vi "fgv_Acq Exited.vi"(8 "error in (no error)":errorcluster, 9 "Function":T1, 11 "Acquisition completed":bool) -> (0 "error out":errorcluster, 3 "Acquisition completed":bool)   [LabVIEW 2020]
uses:
  Typedefs/Read Write Enum.ctl
panel:
  # "SUBROUTINE"
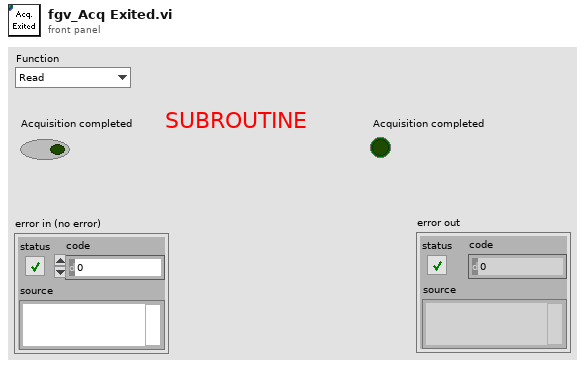
[diagram p1: front panel]
types:
  T1 = typedef "Read Write Enum.ctl" = enum16{"Read", "Write"}
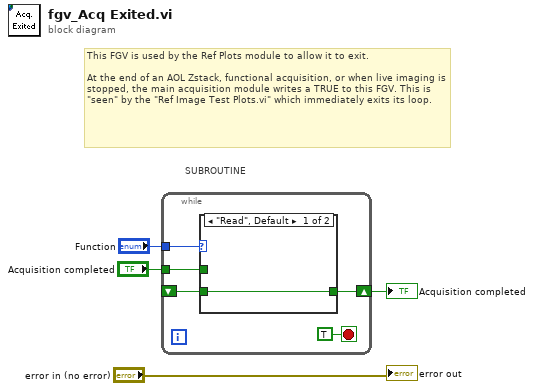
[diagram p0: block diagram]
diagram:
  # "This FGV is used by the Ref Plots module to allow it to exit.\n\nAt the end of an AOL Zstack, functional acquisition, or when live imaging is stopped, the main acquisition module writes a TRUE to this FGV. This is \"seen\" by the \"Ref Image Test Plots.vi\" which immediately exits its loop."
  # "SUBROUTINE"
  n1 = while {
    tunnel: "Function" -> [w8]
    tunnel: "Acquisition completed" -> [w7]
    shift-right: [w6] -> w2
    shift-left: _ -> [w5]
    stop <- TRUE stop-if-true
    n2 = case shown="\"Read\", Default" w8 {
      tunnel: w7 -> [_ w11]
      tunnel: [w10 w11] -> w6
      tunnel: w5 -> [w10 _]
      frame "Read", Default {
      }
      frame "Write" {
      }
    }
  }
  "Acquisition completed" <- w2
  "error out" <- "error in (no error)"
